vi "Get Calibration Method.vi"(7 "ValBufferSize":i32=2048, 8 "error in (no error)":errorcluster {"code" format="%.0x"}, 9 "Port2":i32 format="%.0g", 10 "Port1":i32 format="%.0g", 11 "instrument handle":refnum<k15>) -> (0 "error out":errorcluster {"code" format="%.0x"}, 2 "Val":string, 3 "instrument handle out":refnum<k15>)   [LabVIEW 2014, in "Agilent NA.lvlib"]
doc: "Get Calibration method between 2 specified ports."
uses:
  Agilent NA.lvlib
  AgNA.dll
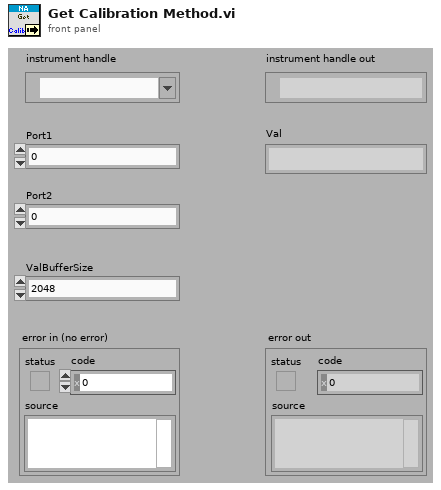
[diagram p1: front panel]
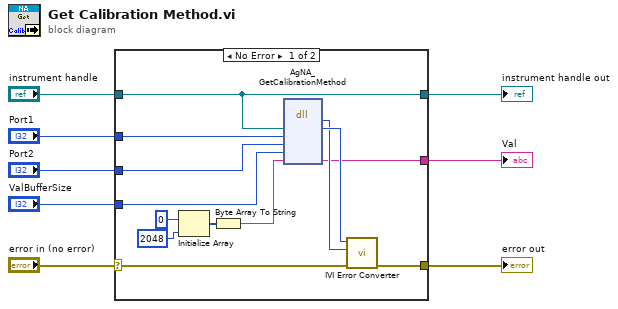
[diagram p0: block diagram]
diagram:
  n1 = case shown="No Error" "error in (no error)" {
    selector: "error in (no error)" -> [w19 w23]
    tunnel: [w18 w23] -> w8
    tunnel: "Port1" -> [w17 _]
    tunnel: "Port2" -> [w16 _]
    tunnel: "ValBufferSize" -> [w15 _]
    tunnel: [w10 _] -> w3
    tunnel: [w9 w22] -> w2
    tunnel: "instrument handle" -> [w9 w22]
    frame No Error {
      n2 = Initialize Array(u8 0 ("element"), 2048 ("dimension size")) -> (w13:u8[])
      n3 = Byte Array To String(unsigned byte array=w13) -> (string=w14:string)
      n4 = dll-call lib="AgNA**.dll" fn="AgNA_GetCalibrationMethod"("Vi"=w9, "Port1"=w17, "Port2"=w16, "ValBufferSize"=w15, "Val"=w14) -> (w20:i32, "Vi"=w21:u32, "Val"=w10:string)  [unwired: 6 in, 2 out]
      n5 = call "IVI Error Converter.vi"("error in (no error)"=w19, "IVI error code (0)"=w20, "instrument handle"=w21) -> ("error out"=w18:errorcluster)  [unwired: 7 in, 1 out]
    }
    frame Error {
    }
  }
  "error out" <- w8
  "instrument handle out" <- w2
  "Val" <- w3
